vi "Server_Data Detection.vi"(8 "error in":errorcluster, 11 "Data":waveform(dbl)) -> (0 "error out":errorcluster, 3 "Warning?":bool)   [LabVIEW 2018, in "Cloud Server.lvlib"]
uses:
  Cloud Server.lvlib
  <vilib>/Analysis/3filter.llb/Elliptic Filter (DBL).vi
  <vilib>/Analysis/NI_AAL_SigProc.lvlib
  <vilib>/Analysis/NI_AALBase.lvlib
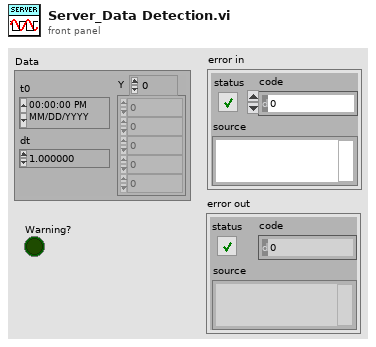
[diagram p1: front panel]
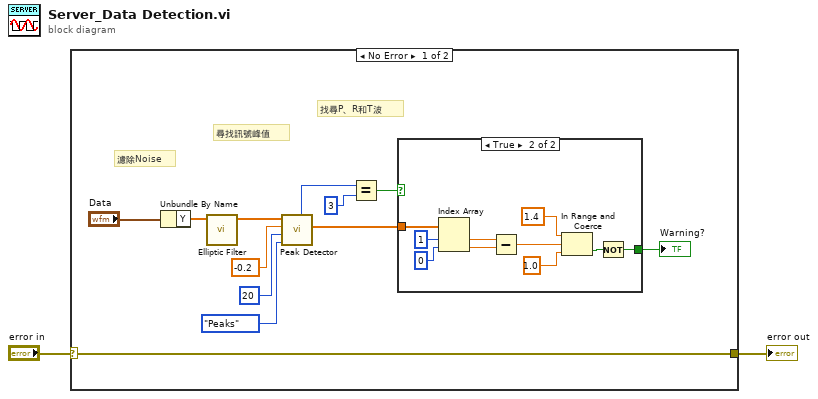
[diagram p0: block diagram]
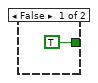
[diagram p2: hidden frame]
diagram:
  n1 = case shown="No Error" "error in" {
    selector: "error in" -> [w3 w26]
    tunnel: [w3 w26] -> w1
    frame No Error {
      # "濾除Noise"
      # "尋找訊號峰值"
      # "找尋P、R和T波"
      n2 = Unbundle By Name("Data") -> ("Y"=w7:dbl[])
      n3 = call-poly <vilib>:"Elliptic Filter.vi"("X"=w7) -> ("Filtered X"=w5:dbl[])  [unwired: 9 in, 1 out]
      n4 = call <vilib>:"Peak Detector.vi"("peaks/valleys"=enum32{"Peaks", "Valleys"}."Peaks", "width"=20, "threshold"=-0.2, "X"=w5) -> ("Amplitudes"=w9:dbl[], "# found"=w12:i32)  [unwired: 3 in, 3 out]
      n5 = Equal?(x=w12, y=3) -> (x = y?=w10:bool)
      n6 = case shown="True" w10 {
        tunnel: [TRUE w16] -> w6
        tunnel: w9 -> [_ w25]
        frame False {
        }
        frame True {
          n7 = Index Array(array=w25, index #1=1 ("index"), index #2=0 ("index")) -> (element #1=w22:dbl, element #2=w21:dbl)
          n8 = Subtract(x=w22, y=w21) -> (x-y=w20:dbl)
          n9 = In Range and Coerce(upper limit=1.4, x=w20, lower limit=1.0) -> (In Range?=w17:bool)  [unwired: 1 out]
          n10 = Not(x=w17) -> (.not. x?=w16:bool)
        }
      }
      "Warning?" <- w6
    }
    frame Error {
    }
  }
  "error out" <- w1
